vi "test_DevicesList.vi"   [LabVIEW 2023]
uses:
  <vilib>/addons/_JKI Toolkits/Caraya/classes/Assert/Assert Not Error.vi
  <vilib>/addons/_JKI Toolkits/Caraya/classes/Assert/Assert Equal Value and Type_Variant.vi
  <vilib>/addons/_JKI Toolkits/Caraya/classes/Test/Test.lvclass
  <vilib>/addons/_JKI Toolkits/Caraya/classes/Assert/Assert.lvclass
  Libraries/DeviceManager/DeviceManager.lvlib
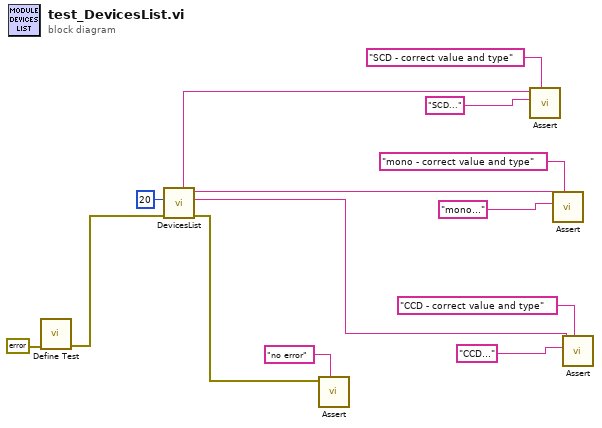
[diagram p0: block diagram]
diagram:
  n1 = call <vilib>:"Define Test.vi"("error in (no error)"=errorcluster {"status"=FALSE, "code"=0, "source"=""}) -> ("error out"=w12:errorcluster)  [unwired: 9 in, 1 out]
  n2 = call "DevicesList.vi"("error in"=w12, "Time out [ms]"=20 ("ID")) -> ("error out"=w11:errorcluster, "CCD-results"=w5:string, "monochromator results"=w4:string, "SCD-results"=w1:string)  [unwired: 5 in, 1 out]
  n3 = call-poly <vilib>:"Assert.vi"("Label"="no error" ("Label (VI Title)"), "Not Error?"=w11) -> ()  [unwired: 8 in, 2 out]
  n4 = call-poly <vilib>:"Assert.vi"("Label"="SCD - correct value and type" ("Label (VI Title)"), "Y"="SCD..." ("Label (VI Title)"), "X"=w1) -> ()  [unwired: 7 in, 2 out]
  n5 = call-poly <vilib>:"Assert.vi"("Label"="mono - correct value and type" ("Label (VI Title)"), "Y"="mono..." ("Label (VI Title)"), "X"=w4) -> ()  [unwired: 7 in, 2 out]
  n6 = call-poly <vilib>:"Assert.vi"("Label"="CCD - correct value and type" ("Label (VI Title)"), "Y"="CCD..." ("Label (VI Title)"), "X"=w5) -> ()  [unwired: 7 in, 2 out]
